vi "2_wavelength_subVI - Copy.vi"() -> (0 "Intensity_2":dbl[](array[numeric]), 1 "Intensity_1":dbl[](array[numeric]), 2 "Wavelength_2":dbl[](array[numeric]), 3 "Wavelength_1":dbl[](array[numeric]))   [LabVIEW 2018]
uses:
  <vilib>/Utility/file.llb/Read Delimited Spreadsheet (DBL).vi
panel:
  in  "file path (dialog if empty)":path
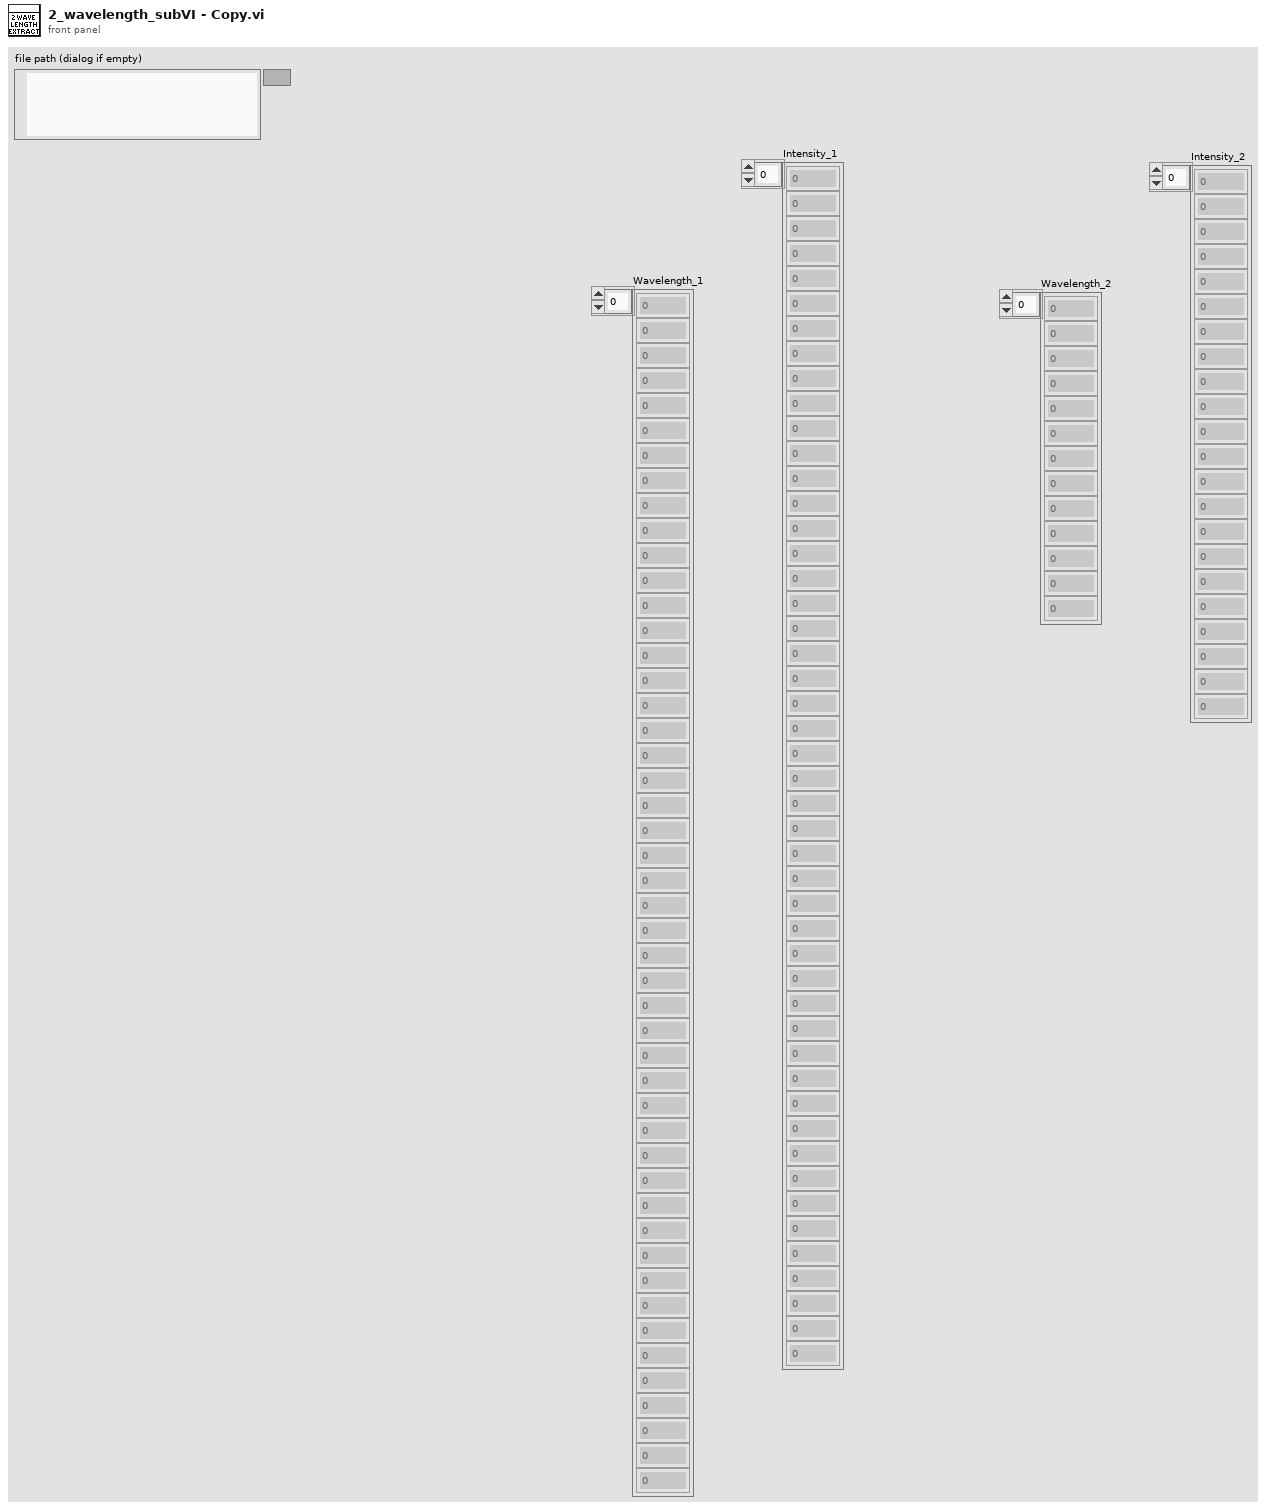
[diagram p1: front panel]
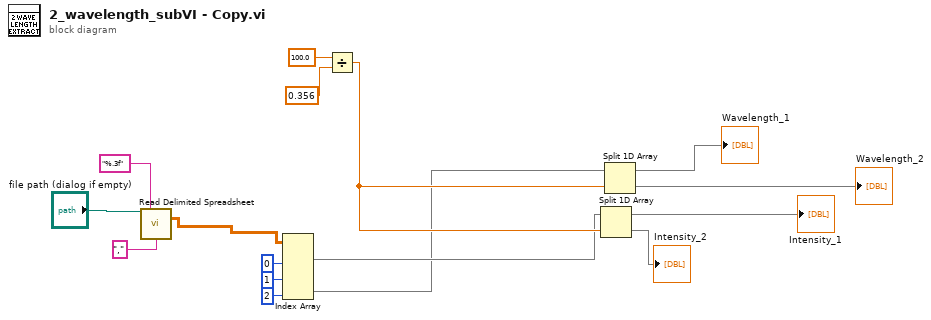
[diagram p0: block diagram]
diagram:
  n1 = call-poly <vilib>:"Read Delimited Spreadsheet.vi"("file path (dialog if empty)"="file path (dialog if empty)", "format (%.3f)"="%.3f", "delimiter (\\t)"="," ("delimiter (\\t)")) -> ("all rows"=w8:dbl[][])  [unwired: 7 in, 5 out]
  n2 = Index Array(array=w8, index (col) #1=0 ("disabled index (col)"), index (col) #2=1 ("index (col)"), index (col) #3=2 ("index (col)")) -> (element #1=w4:dbl[], element #3=w3:dbl[])  [unwired: 3 in, 1 out]
  n3 = Divide(x=100.0, y=0.356) -> (x/y=w14:dbl)
  n4 = Split 1D Array(array=w4, index=w14) -> (first subarray=→"Intensity_1":dbl[], second subarray=→"Intensity_2":dbl[])
  n5 = Split 1D Array(array=w3, index=w14) -> (first subarray=→"Wavelength_1":dbl[], second subarray=→"Wavelength_2":dbl[])
